vi "Get Item Property (Path).vi"(8 "error in (no error)":errorcluster, 9 "Default Value":path, 10 "Property Name":string, 11 "Item Ref in":T1 format="%.0x") -> (0 "error out":errorcluster, 1 "Value":path, 3 "Item Ref out":T1 format="%.0x", 4 "Found?":bool)   [LabVIEW 2020, in "Custom Device API.lvlib"]
doc: "Returns the <B>Value</B> of a specific item <B>Property Name</B>. Properties do not inherit within a custom device, so <B>Item Ref in</B> must reference the specific item on which the property is set. \n\nFor instances with a <B>Default Value</B> input, the <B>Value</B> output returns this value if the <B>Property Name</B> is not found for the specified item. Wire data to the <B>Default Value</B> input to determine the polymorphic instance to use or manually select the instance."
uses:
  <vilib>/NI VeriStand/Custom Device API/Custom Device API.lvlib
  <vilib>/NI VeriStand/Custom Device API/Custom Device Item Ref.ctl
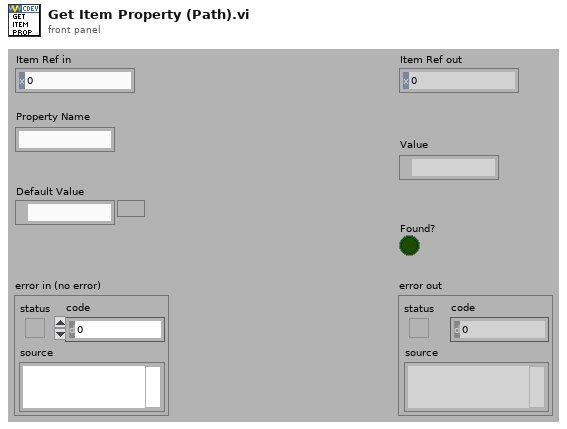
[diagram p1: front panel]
types:
  T1 = typedef "Custom Device API.lvlib/Custom Device Item Ref.ctl" = u64
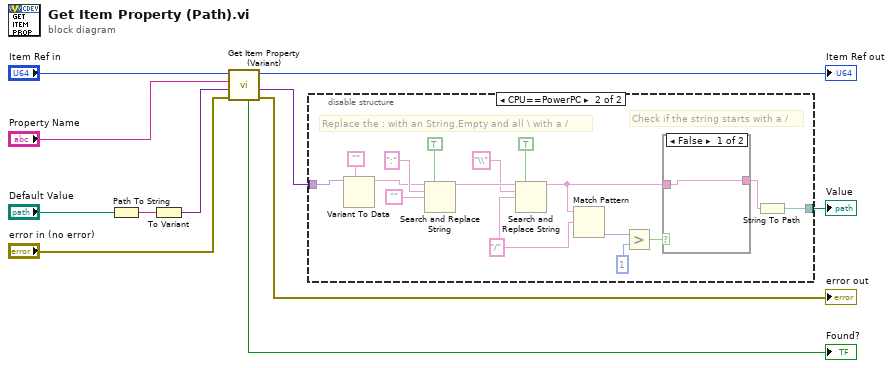
[diagram p0: block diagram]
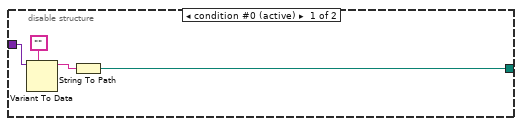
[diagram p2: hidden frame]
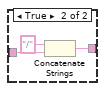
[diagram p3: hidden frame]
diagram:
  n1 = Path To String(path="Default Value") -> (string=w2:string)
  n2 = To Variant(anything=w2) -> (Variant=w7:variant)
  n3 = call <vilib>:"Get Item Property (Variant).vi"("error in (no error)"="error in (no error)", "Default Value"=w7, "Property Name"="Property Name", "Item Ref in"="Item Ref in") -> ("error out"=→"error out":errorcluster, "Value"=w4:variant, "Item Ref out"=→"Item Ref out":T1, "Found?"=→"Found?":bool)  [unwired: 4 out]
  n4 = disable-structure shown="CPU==PowerPC" {
    disable-tunnel: w4 -> [w14 w20]
    disable-tunnel: [w12 w17] -> w1
    frame condition #0 (active) {
      n5 = Variant To Data(type="", Variant=w14) -> (data=w15:string)  [unwired: 1 in, 1 out]
      n6 = String To Path(string=w15) -> (path=w12:path)
    }
    frame condition #1 {
      w31 = "/" ("replace string (\"\")")
      # "Check if the string starts with a /"
      # "Replace the : with an String.Empty and all \\ with a /"
      n7 = Variant To Data(type="", Variant=w20) -> (data=w22:string)  [unwired: 1 in, 1 out]
      n8 = Search and Replace String(replace all?=TRUE ("replace all? (F)"), input string=w22, search string=":", replace string="") -> (result string=w27:string)  [unwired: 4 in, 3 out]
      n9 = Search and Replace String(replace all?=TRUE ("replace all? (F)"), input string=w27, search string="\\", replace string=w31) -> (result string=w19:string)  [unwired: 4 in, 3 out]
      n10 = Match Pattern(string=w19, regular expression=w31) -> (offset past match=w28:i32)  [unwired: 1 in, 3 out]
      n11 = Greater?(x=w28, y=1) -> (0:w30:bool)
      n12 = case shown="False" w30 {
        tunnel: w19 -> [w32 w35]
        tunnel: [w32 w33] -> w18
        frame False {
        }
        frame True {
          n13 = Concatenate Strings("/" ("string"), w35) -> (w33:string)
        }
      }
      n14 = String To Path(string=w18) -> (path=w17:path)
    }
  }
  "Value" <- w1
